vi "RemoveGear mods.vi"(1 "xbox data":cluster{"Open/":bool, "Middle ":bool}) -> ()   [LabVIEW 2016]
panel:
  in  "Close Angle Left":dbl
  in  "Close Angle Right":dbl
  in  "Middle Angle Left":dbl
  in  "Middle Angle Right":dbl
  in  "Open Angle Left":dbl
  in  "Open Angle Right":dbl
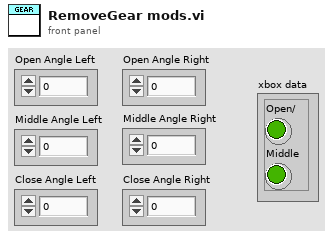
[diagram p1: front panel]
types:
  T1 = typedef "WPI_ServoDeviceRef.ctl" = cluster{"DeviceStatus":errorcluster, "PWM Channel":T2, "DeadBand":T3}
  T2 = typedef "FPGA_DIOPWMChannel.ctl" = enum8{"PWM 0", "PWM 1", "PWM 2", "PWM 3", "PWM 4", "PWM 5", "PWM 6", "PWM 7", "PWM 8", "PWM 9", "PWM MXP 0", "PWM MXP 1", "PWM MXP 2", "PWM MXP 3", "PWM MXP 4", "PWM MXP 5", "PWM MXP 6", "PWM MXP 7", "PWM MXP 8", "PWM MXP 9", "Invalid"}
  T3 = typedef "WPI_PWMDeadband.ctl" = cluster{"Name":string, "maxPositivePwm":i32, "minPositivePwm":i32, "centerPwm":i32, "maxNegativePwm":i32, "minNegativePwm":i32, "angularRange":u16}
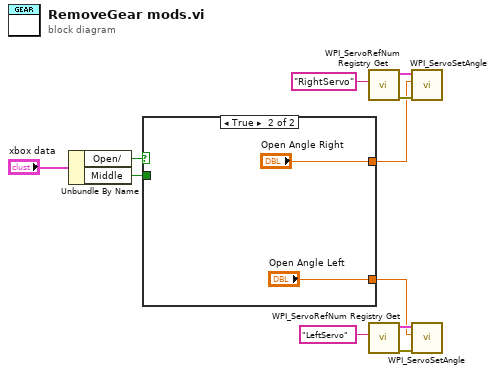
[diagram p0: block diagram]
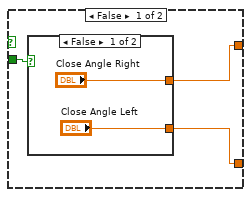
[diagram p2: hidden frame]
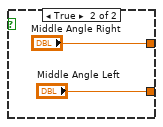
[diagram p3: hidden frame]
diagram:
  n1 = Unbundle By Name("xbox data") -> ("Open/"=w10:bool, "Middle"=w1:bool)
  n2 = case shown="True" w10 {
    tunnel: [w13 "Open Angle Right"] -> w3
    tunnel: [w12 "Open Angle Left"] -> w2
    tunnel: w1 -> [w14 _]
    frame False {
      n3 = case shown="False" w14 {
        tunnel: ["Close Angle Left" "Middle Angle Left"] -> w12
        tunnel: ["Close Angle Right" "Middle Angle Right"] -> w13
        frame False {
        }
        frame True {
        }
      }
    }
    frame True {
    }
  }
  n4 = call <vilib>:"WPI_ServoRefNum Registry Get.vi"("refnum name"="RightServo") -> ("error out"=w7:errorcluster, "ServoDeviceRef"=w6:T1)  [unwired: 9 in]
  n5 = call <vilib>:"WPI_ServoRefNum Registry Get.vi"("refnum name"="LeftServo") -> ("error out"=w4:errorcluster, "ServoDeviceRef"=w5:T1)  [unwired: 9 in]
  n6 = call <vilib>:"WPI_ServoSetAngle.vi"("error in (no error)"=w7, "Angle"=w3, "ServoDeviceRef"=w6) -> ()  [unwired: 7 in, 2 out]
  n7 = call <vilib>:"WPI_ServoSetAngle.vi"("error in (no error)"=w4, "Angle"=w2, "ServoDeviceRef"=w5) -> ()  [unwired: 7 in, 2 out]
